vi "Day 2.vi"() -> ()   [LabVIEW 2019]
panel:
  out "Common Characters":string
  out "Box 2":string
  out "Box 1":string
  out "Error Out":errorcluster
  out "Checksum":i32
  out "Triples":i32
  out "Doubles":i32
  in  "Error In":errorcluster
  in  "Relative Path to Raw Data":string="Day 2\\Day 2 Raw Input.txt"
  # "Part 2"
  # "Part 1"
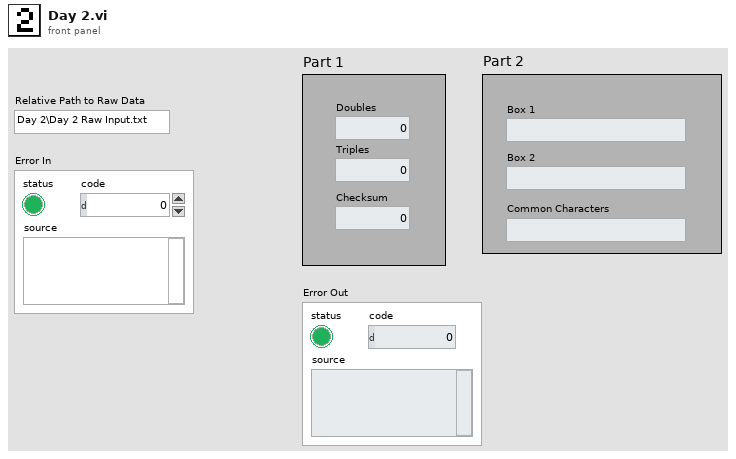
[diagram p1: front panel]
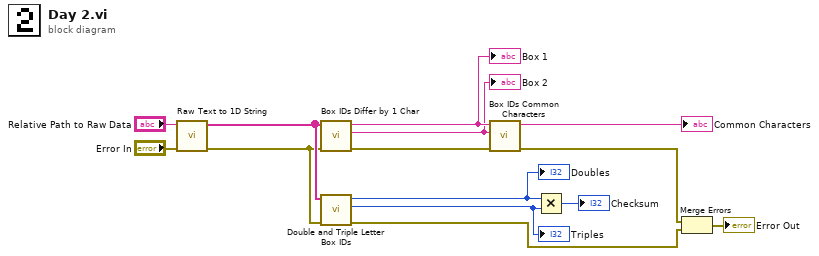
[diagram p0: block diagram]
diagram:
  n1 = call "Raw Text to 1D String.vi"("Error In"="Error In", "Relative Path to Input File"="Relative Path to Raw Data") -> ("Error Out"=w8:errorcluster, "1D String Array"=w9:string[])  [unwired: 8 in]
  n2 = call "Box IDs Differ by 1 Char.vi"("Error In"=w8, "1D String Array"=w9) -> ("Error Out"=w2:errorcluster, "Box 2"=w4:string, "Box 1"=w5:string)  [unwired: 7 in]
  "Box 1" <- w5
  "Box 2" <- w4
  n3 = call "Double and Triple Letter Box IDs.vi"("Error In"=w8, "1D String Array"=w9) -> ("Error Out"=w7:errorcluster, "Triples"=w11:i32, "Doubles"=w12:i32)  [unwired: 7 in]
  "Doubles" <- w12
  "Triples" <- w11
  n4 = call "Box IDs Common Characters.vi"("Error In"=w2, "Box in"=w4, "Box 1"=w5) -> ("Error Out"=w1:errorcluster, "Common Characters"=→"Common Characters":string)  [unwired: 7 in]
  n5 = Multiply(x=w12, y=w11) -> (x*y=→"Checksum":i32)
  n6 = Merge Errors(w1, w7) -> (→"Error Out":errorcluster)
